vi "Untitled 1.vi"() -> ()   [LabVIEW 2019]
panel:
  out "Waveform Chart":dbl(graph)
  in  "stop":bool
  in  "Kasuj":bool
  in  "C":bool
  in  "B":bool
  in  "A":bool
  out "String":string
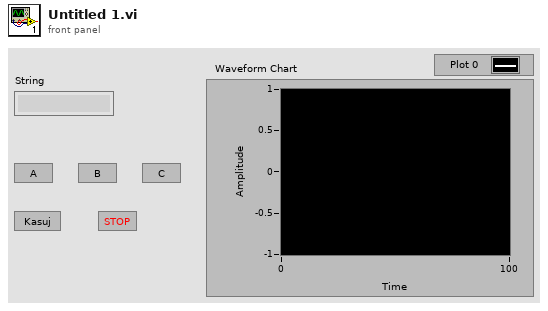
[diagram p1: front panel]
types:
  T1 = typedef "eventsource.ctl" = u32
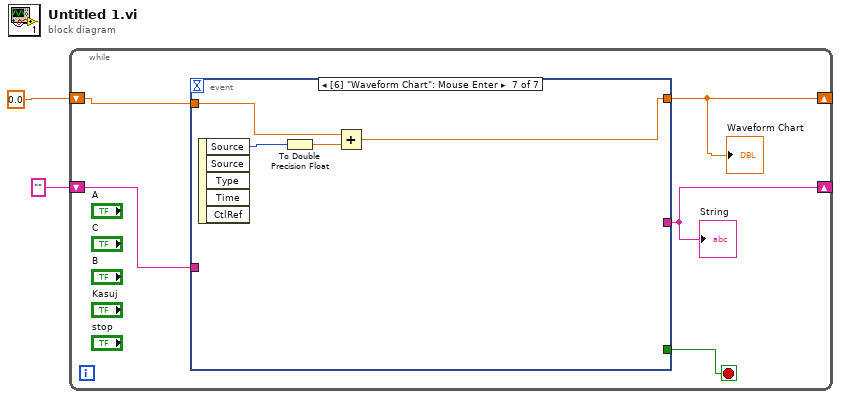
[diagram p0: block diagram]
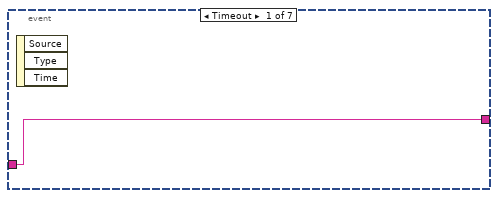
[diagram p2: hidden frame]
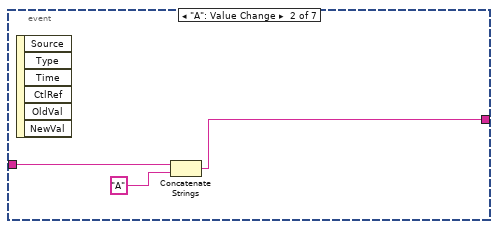
[diagram p3: hidden frame]
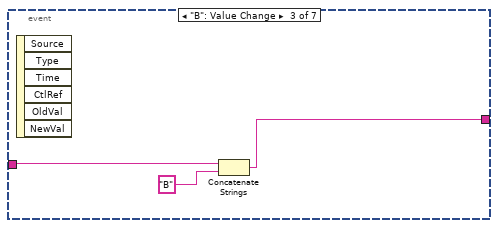
[diagram p4: hidden frame]
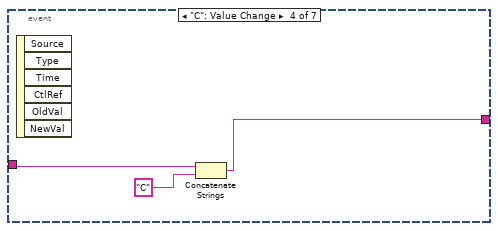
[diagram p5: hidden frame]
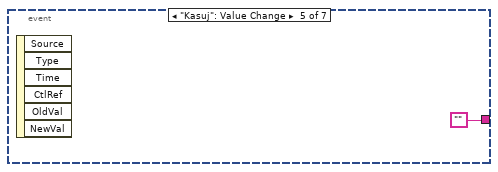
[diagram p6: hidden frame]
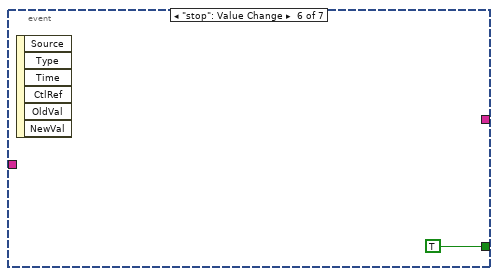
[diagram p7: hidden frame]
diagram:
  n1 = while {
    shift-right: [w6] -> _
    shift-left: "" -> [w7]
    shift-right: [w4] -> _
    shift-left: 0.0 ("Waveform Chart") -> [w3]
    stop <- w5 stop-if-true
    n2 = event shown="[6] \"Waveform Chart\": Mouse Enter" {
      selector: _ -> [_ _ _ _ _ _ _]
      dyn-events: _ -> [_ _ _ _ _ _ _]
      timeout: _ -> [_ _ _ _ _ _ _]
      tunnel: w7 -> [w8 w11 w13 w16 _ _ _]
      tunnel: [w8 w9 w12 w15 "" _ _] -> w6
      tunnel: [_ _ _ _ _ TRUE _] -> w5
      tunnel: [_ _ _ _ _ _ w20] -> w4
      tunnel: w3 -> [_ _ _ _ _ _ w21]
      event Timeout {
        n3 = event-data() -> ()  [unwired: 1 in, 3 out]
      }
      event "A": Value Change {
        n4 = event-data() -> ()  [unwired: 1 in, 6 out]
        n5 = Concatenate Strings(w11, "A" ("string")) -> (w9:string)
      }
      event "B": Value Change {
        n6 = event-data() -> ()  [unwired: 1 in, 6 out]
        n7 = Concatenate Strings(w13, "B" ("string")) -> (w12:string)
      }
      event "C": Value Change {
        n8 = event-data() -> ()  [unwired: 1 in, 6 out]
        n9 = Concatenate Strings(w16, "C" ("string")) -> (w15:string)
      }
      event "Kasuj": Value Change {
        n10 = event-data() -> ()  [unwired: 1 in, 6 out]
      }
      event "stop": Value Change {
        n11 = event-data() -> ()  [unwired: 1 in, 6 out]
      }
      event "Waveform Chart": Mouse Enter {
        n12 = event-data() -> ("Source"=w23:T1)  [unwired: 1 in, 4 out]
        n13 = To Double Precision Float(number=w23) -> (double precision float=w22:dbl)
        n14 = Add(x=w21, y=w22) -> (x+y=w20:dbl)
      }
    }
    "String" <- w6
    "Waveform Chart" <- w4
  }
